vi "Go To Temperature.vi"(8 "error in (no error)":errorcluster, 9 "Target Temperature Rate (K/min)":dbl, 10 "Target Temperature (K)":dbl, 11 "instrument.PPMS2 in":refnum<class "instrument.PPMS2.lvclass">) -> (0 "error out":errorcluster, 3 "instrument.PPMS2 out":refnum<class "instrument.PPMS2.lvclass">)   [LabVIEW 2016, in "instrument.PPMS2.lvclass"]
uses:
  instrument.PPMS2.lvclass
  PPMS Global.vi
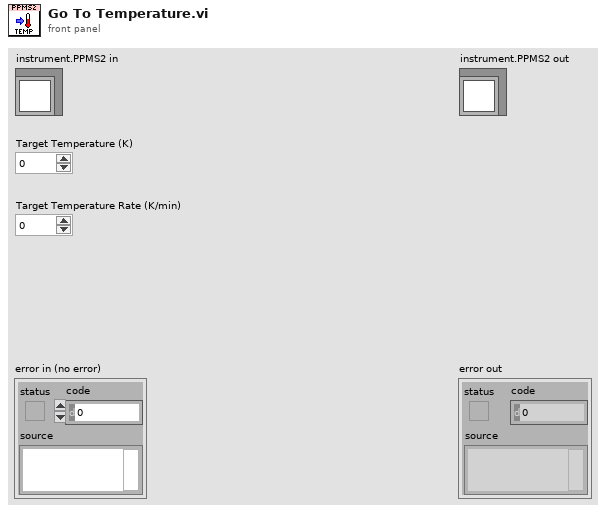
[diagram p1: front panel]
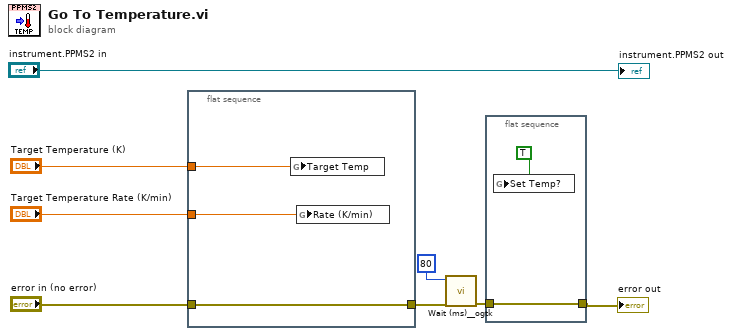
[diagram p0: block diagram]
diagram:
  n1 = flat-sequence {
    tunnel: "error in (no error)" -> [w11]
    tunnel: [w11] -> w6
    tunnel: "Target Temperature (K)" -> [w10]
    tunnel: "Target Temperature Rate (K/min)" -> [w9]
    frame #0 {
      n2 = global write "PPMS Global.vi" "Target Temp"(w10) -> ()
      n3 = global write "PPMS Global.vi" "Rate (K/min)"(w9) -> ()
    }
  }
  n4 = call <userlib>:"Wait (ms)__ogtk.vi"("error in (no error)"=w6, "milliseconds to wait"=u32 80) -> ("error out"=w8:errorcluster)  [unwired: 8 in, 1 out]
  n5 = flat-sequence {
    tunnel: w8 -> [w12]
    tunnel: [w12] -> w5
    frame #0 {
      n6 = global write "PPMS Global.vi" "Set Temp?"(TRUE ("Set Field?")) -> ()
    }
  }
  "error out" <- w5
  "instrument.PPMS2 out" <- "instrument.PPMS2 in"
